vi "Task Stop.vi"(8 "error in (no error)":errorcluster, 11 "VolatusCoreTask in":refnum<class "VolatusCoreTask.lvclass">) -> (0 "error out":errorcluster, 3 "VolatusCoreTask out":refnum<class "VolatusCoreTask.lvclass">)   [LabVIEW 2020, in "Volatus.lvlib" / "VolatusCoreTask.lvclass"]
uses:
  VolatusCoreTask.lvclass
  VolatusCoreTask.lvclass/VolatusCoreTask.ctl
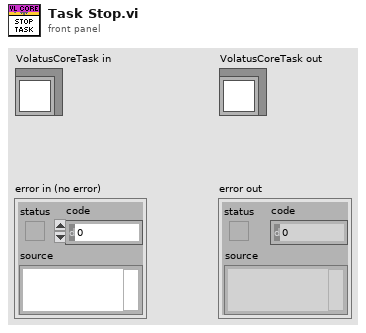
[diagram p1: front panel]
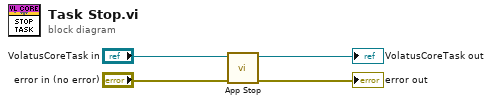
[diagram p0: block diagram]
diagram:
  n1 = call "App Stop.vi"("error in (no error)"="error in (no error)", "VolatusCoreTask in"="VolatusCoreTask in") -> ("error out"=→"error out":errorcluster, "VolatusCoreTask out"=→"VolatusCoreTask out":refnum<class "VolatusCoreTask.lvclass">)  [unwired: 8 in]
